vi "SQLite Get Calibration Kb Array.vi"(7 "Main":string="0", 8 "error in (no error)":errorcluster, 11 "VariableName":string) -> (0 "error out":errorcluster, 1 "Calibration Unit":T4, 2 "Calibration":T1, 3 "Calibration Kb&Volts":T2, 4 "XY":cluster{"X":dbl[], "Y":dbl[]}, 5 "Result Set 2":string[][](table) caption="Result Set (from first statement with results)", 6 "number":dbl[][](array[numeric]))   [LabVIEW 2017, in "SQLite.lvclass"]
doc: "从数据库读取多点校准数据，自动计算Kb的值。\n2015-11-03 15:56:09\n蒋松\njiangsong@outlook.com"
uses:
  SQLite.lvclass
  Calibration Unit.ctl
  Calibration Kb and Volt.ctl
  Calibration K and b Array.ctl
  Calibration K and b.ctl
  SQLiteFileName.ctl
  TabelFullName.ctl
  <vilib>/Utility/error.llb/Trim Whitespace.vi
  <userlib>/_MGI/1D Array/MGI Calculate Array Differences/MGI Calculate Array Differences (DBL[]).vi
  <userlib>/LabSQL/LabSQL.lvlib
  <userlib>/sushu/sushu.lvlib
panel:
  out "Select SQL CMD":string
  in  "error in (no error) 2":errorcluster
  out "y(i)=x(i)-x(i-1) 2":dbl[](array[numeric]) format="%.2f"
  out "y(i)=x(i)-x(i-1)":dbl[](array[numeric]) format="%.2f"
  out "x/y":dbl[](array[numeric])
  in  "OK":bool
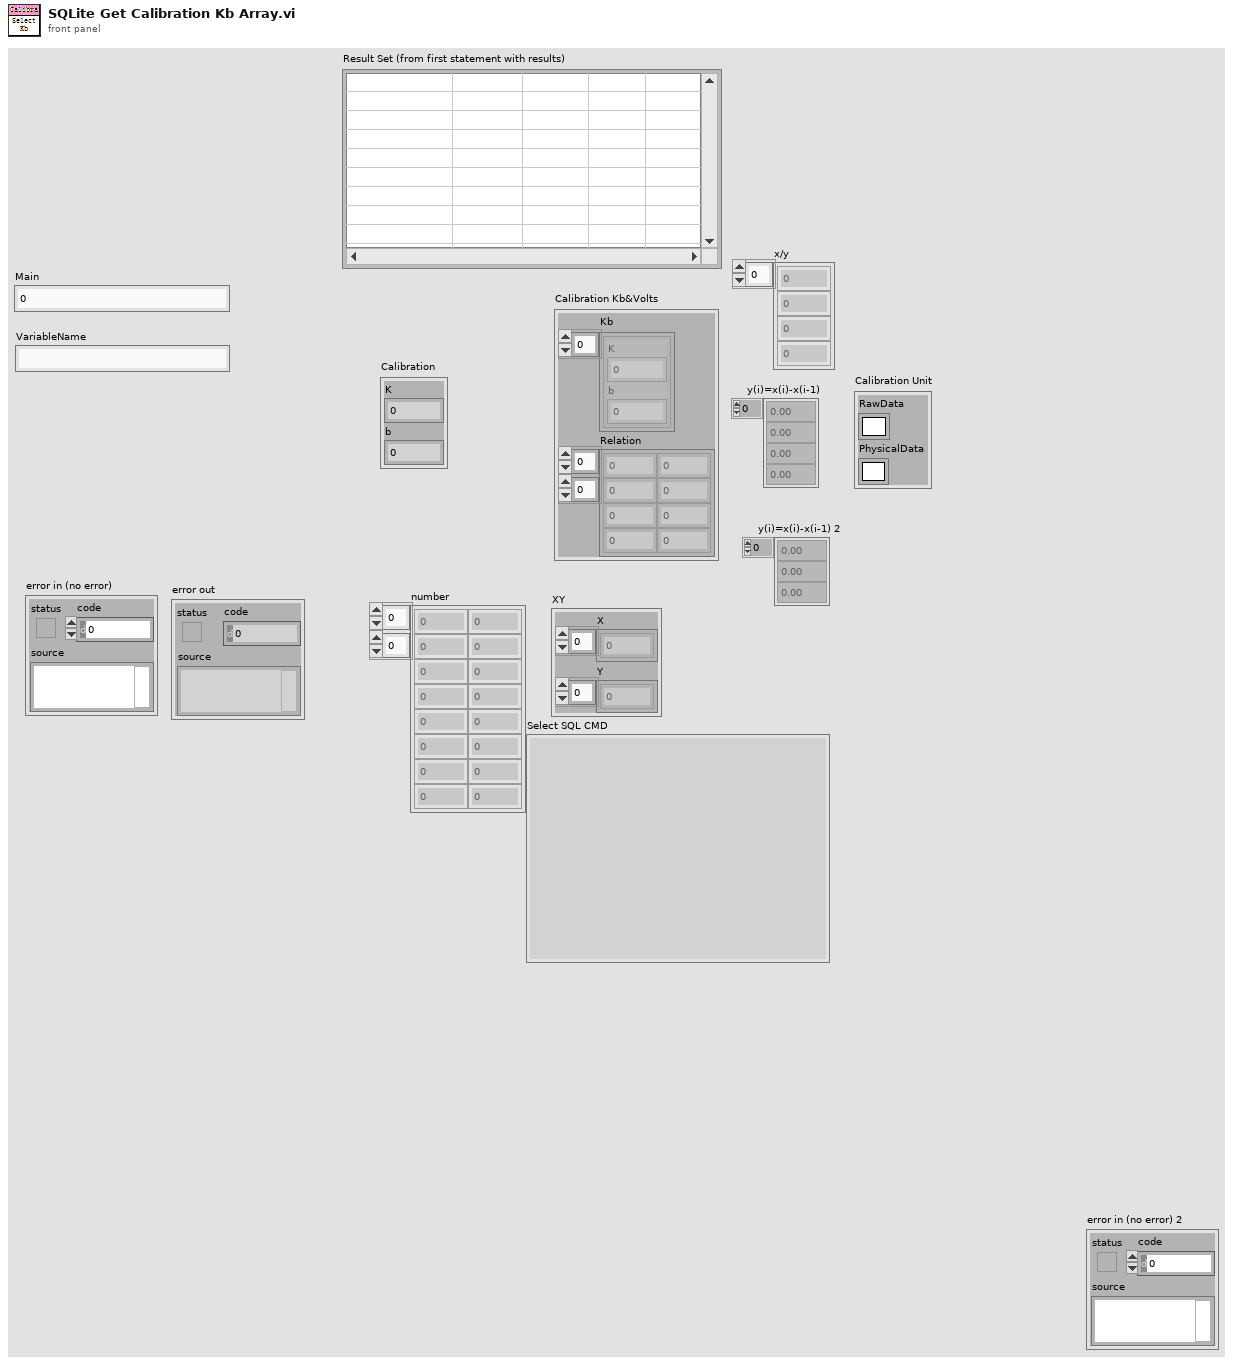
[diagram p1: front panel]
types:
  T1 = typedef "SQLite.lvclass/Calibration K and b.ctl" = cluster{"K":dbl, "b":dbl}
  T2 = typedef "SQLite.lvclass/Calibration Kb and Volt.ctl" = cluster{"Kb":T3, "Relation":dbl[][]}
  T3 = typedef "SQLite.lvclass/Calibration K and b Array.ctl" = T1[]
  T4 = typedef "SQLite.lvclass/Calibration Unit.ctl" = cluster{"RawData":string, "PhysicalData":string}
  T5 = typedef "SQLite.lvclass/TabelFullName.ctl" = string
  T6 = typedef "SQLite.lvclass/SQLiteFileName.ctl" = string
  T7 = enum16{"Other", "SQL2008", "SQLite", "Access", "MySQL"}
  T8 = cluster{"Current VI Reference":refnum<vi>, "Close Panel on Exit?":bool}
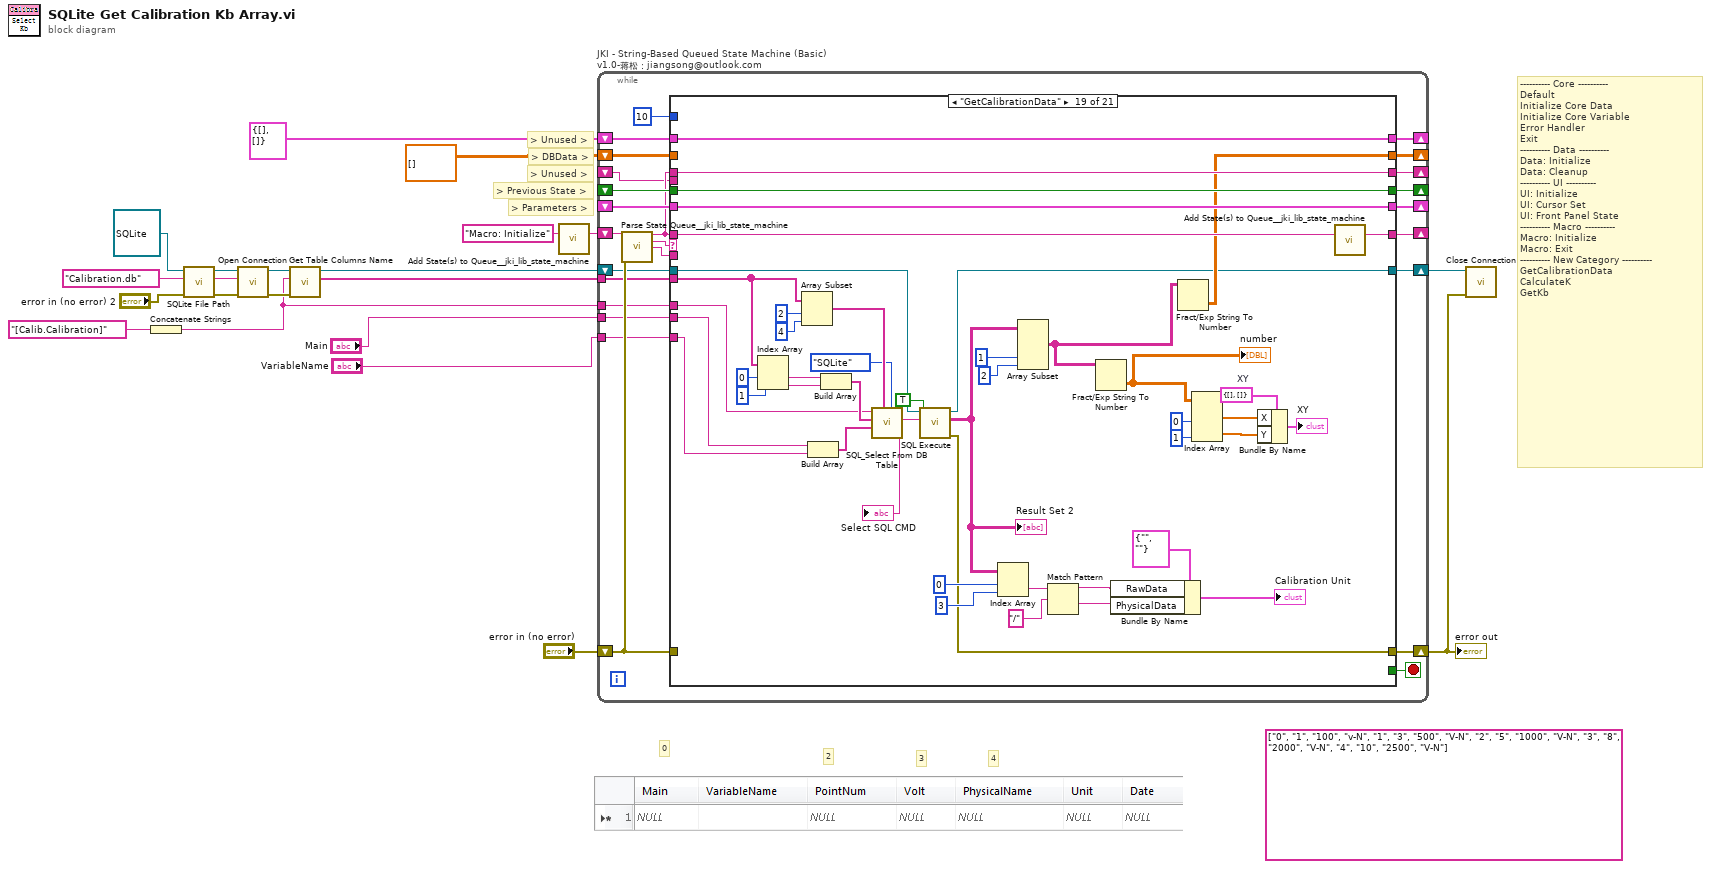
[diagram p0: block diagram]
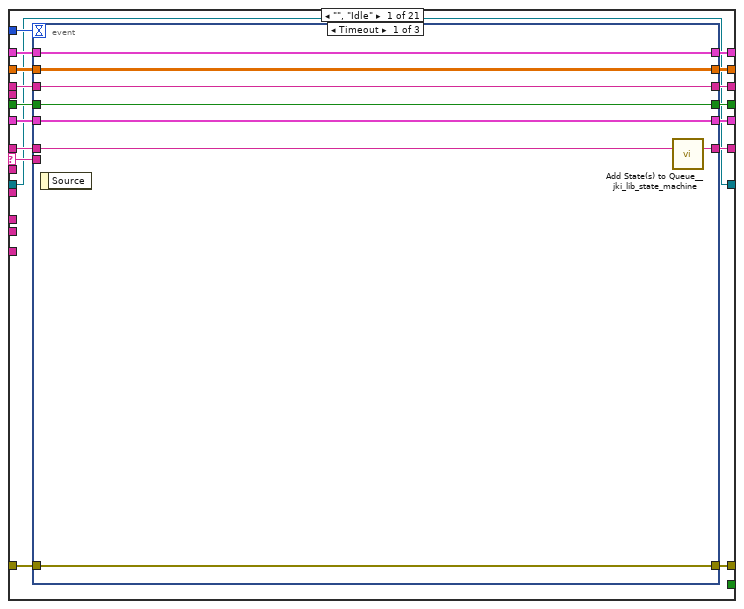
[diagram p2: hidden frame]
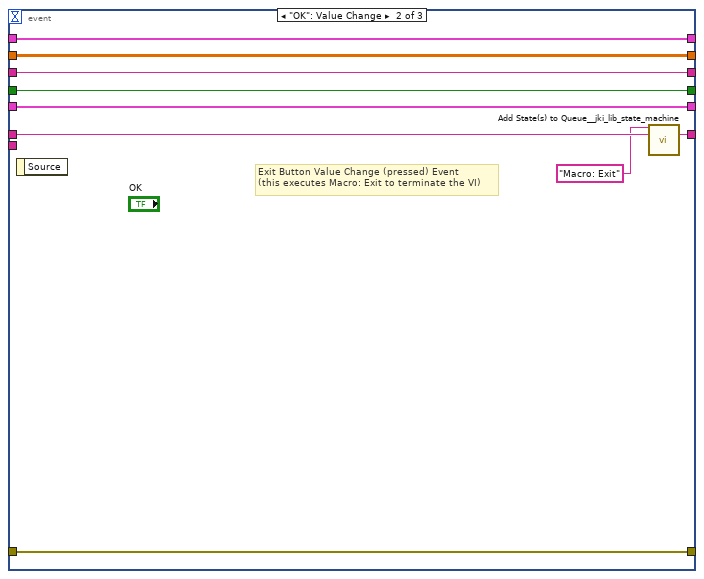
[diagram p3: hidden frame]
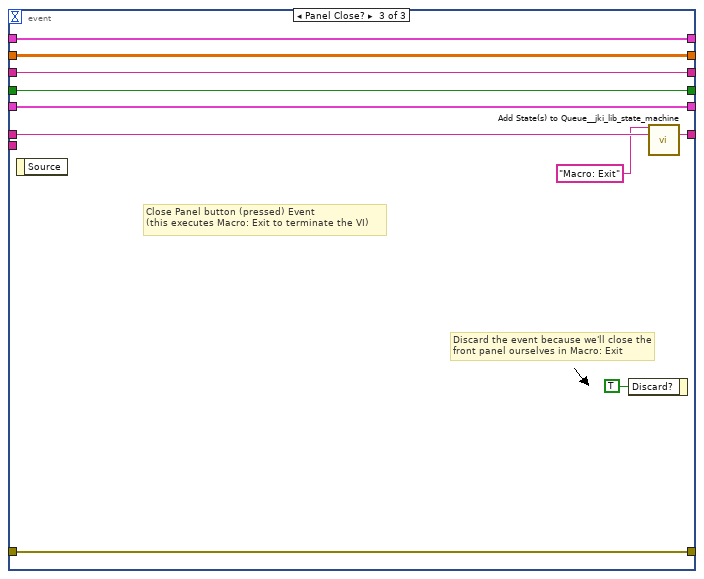
[diagram p4: hidden frame]
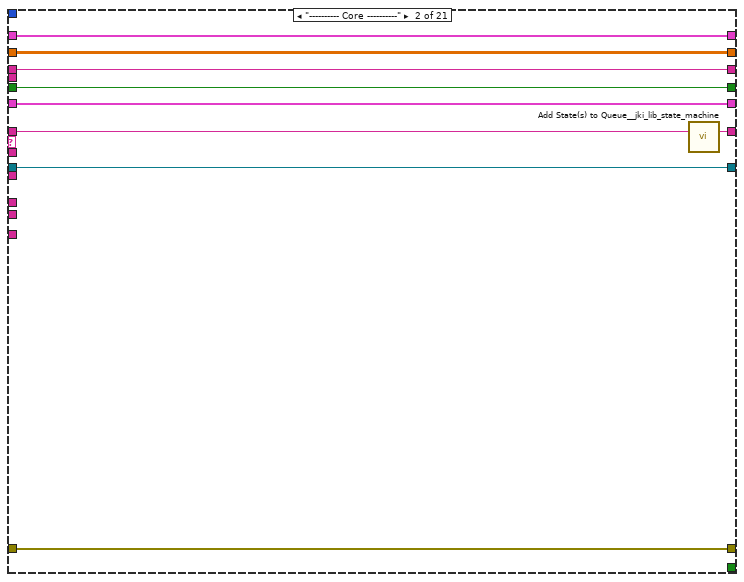
[diagram p5: hidden frame]
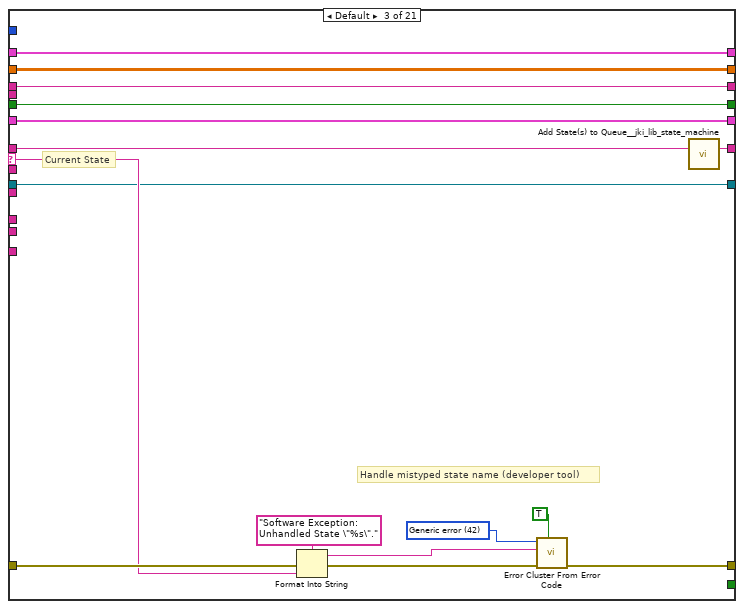
[diagram p6: hidden frame]
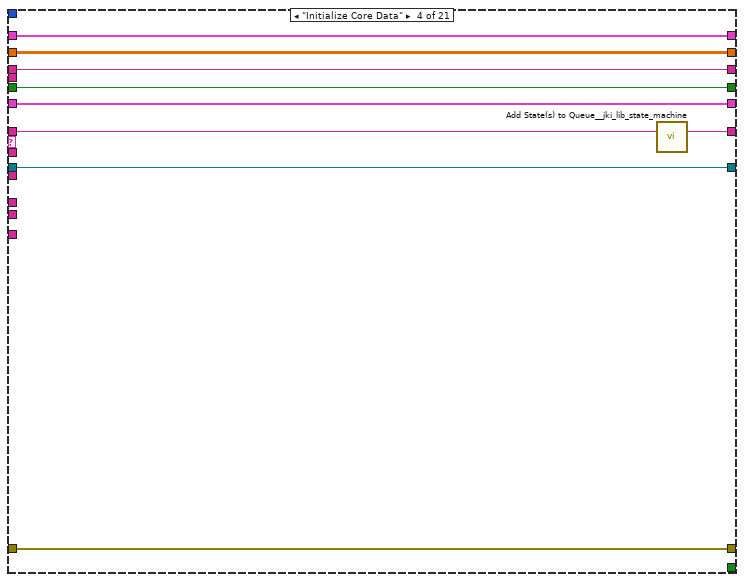
[diagram p7: hidden frame]
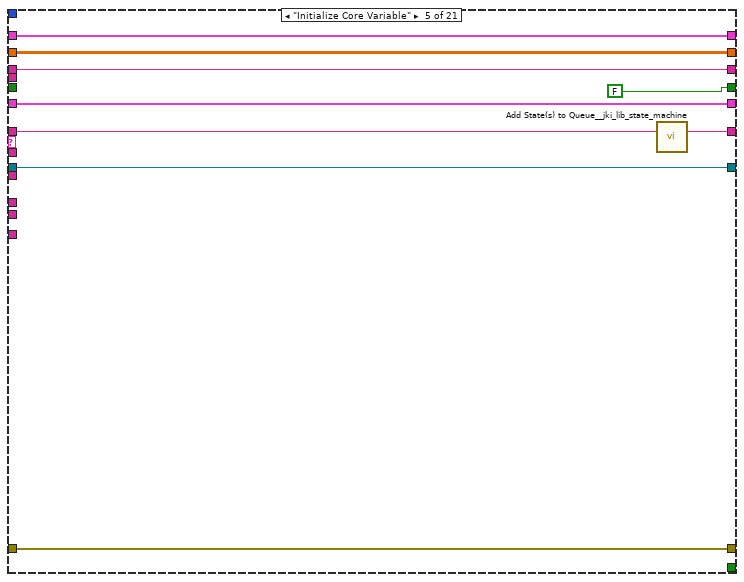
[diagram p8: hidden frame]
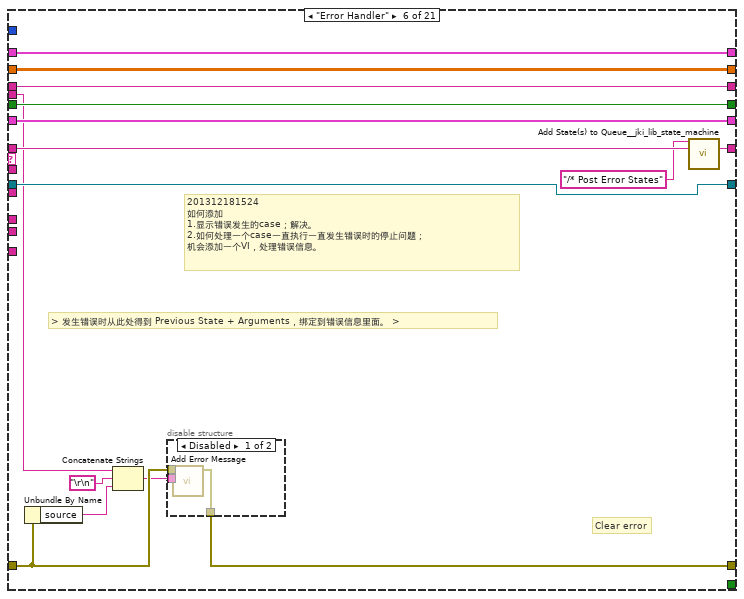
[diagram p9: hidden frame]
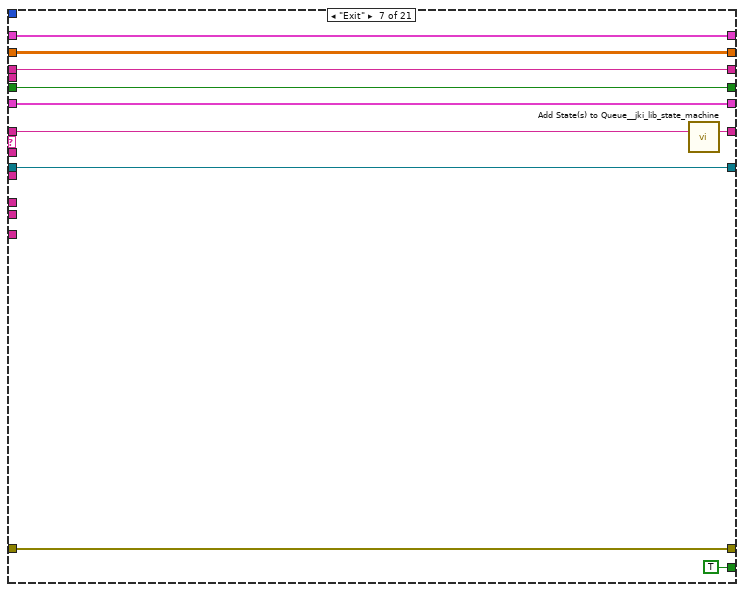
[diagram p11: hidden frame]
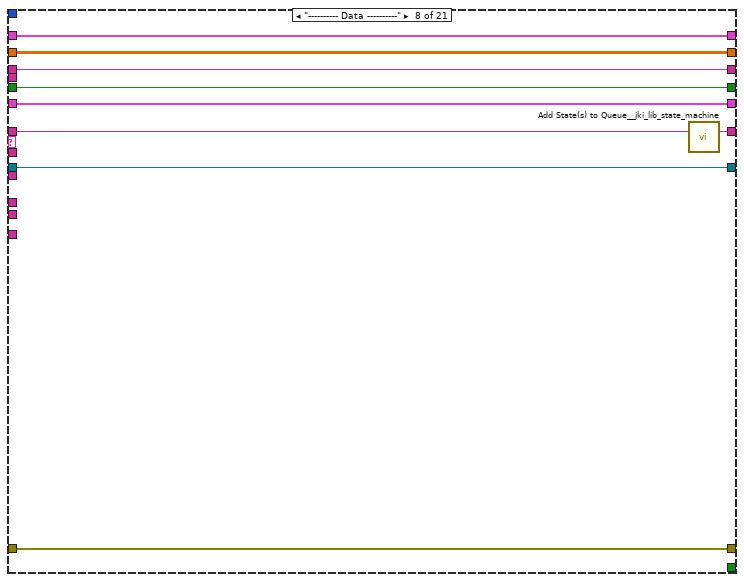
[diagram p12: hidden frame]
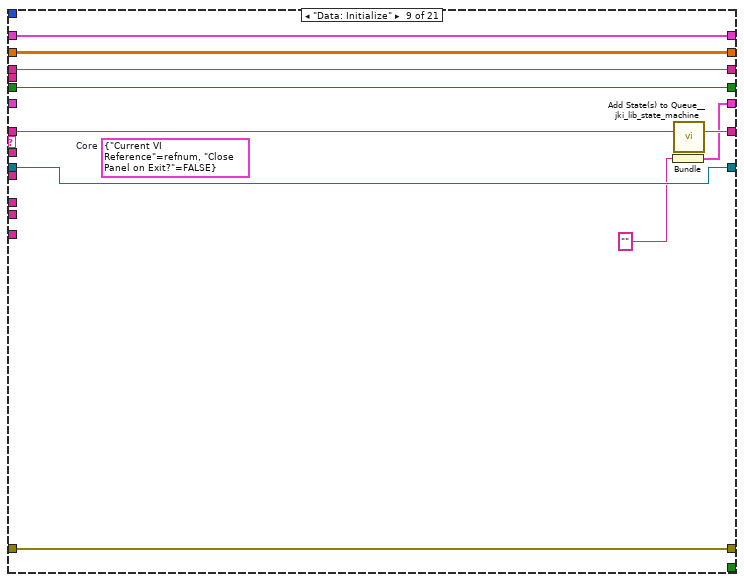
[diagram p13: hidden frame]
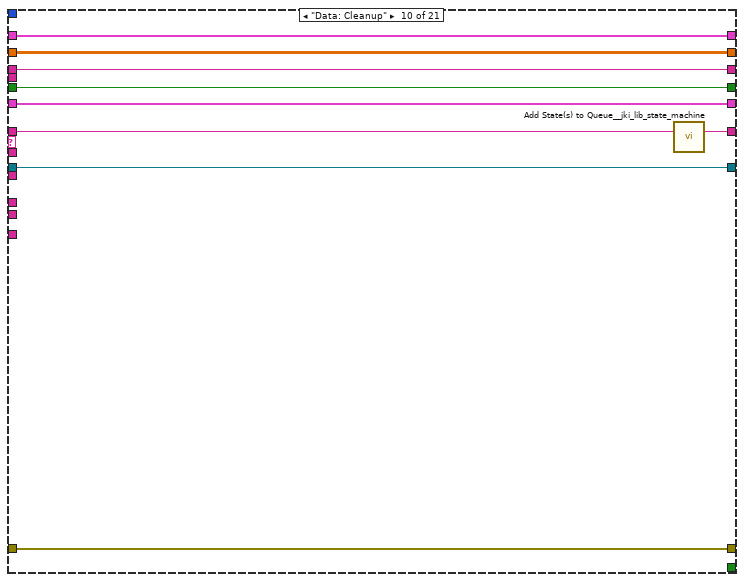
[diagram p14: hidden frame]
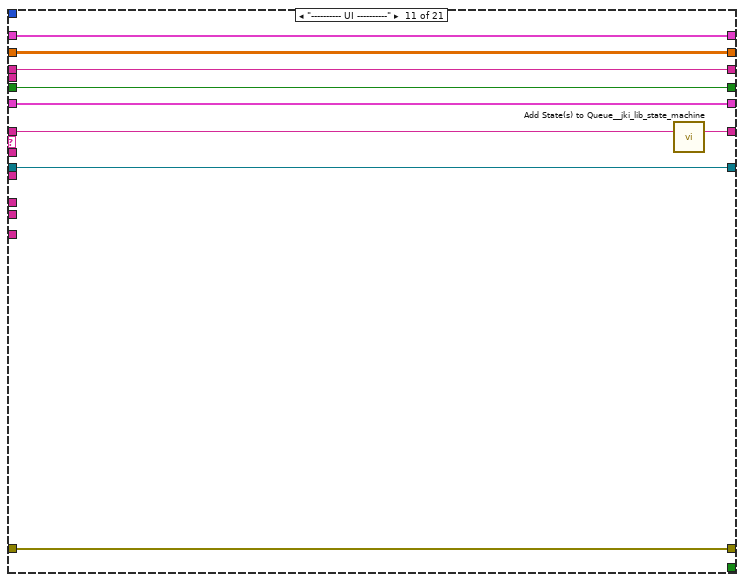
[diagram p15: hidden frame]
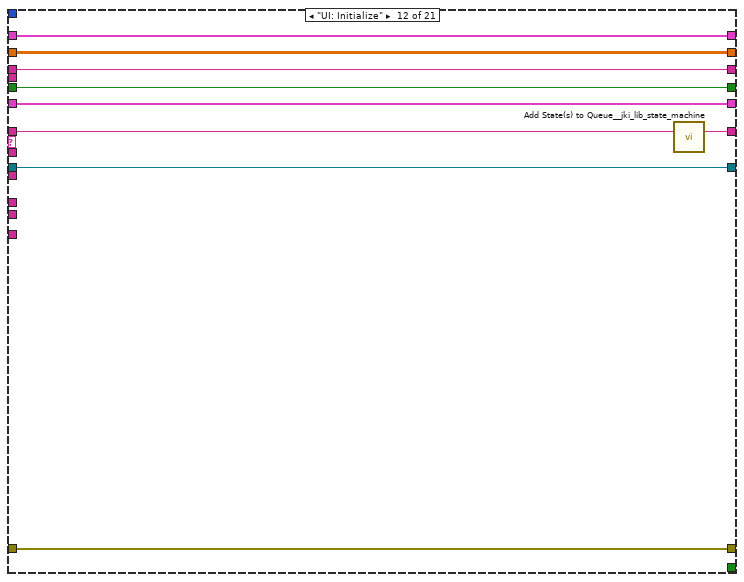
[diagram p16: hidden frame]
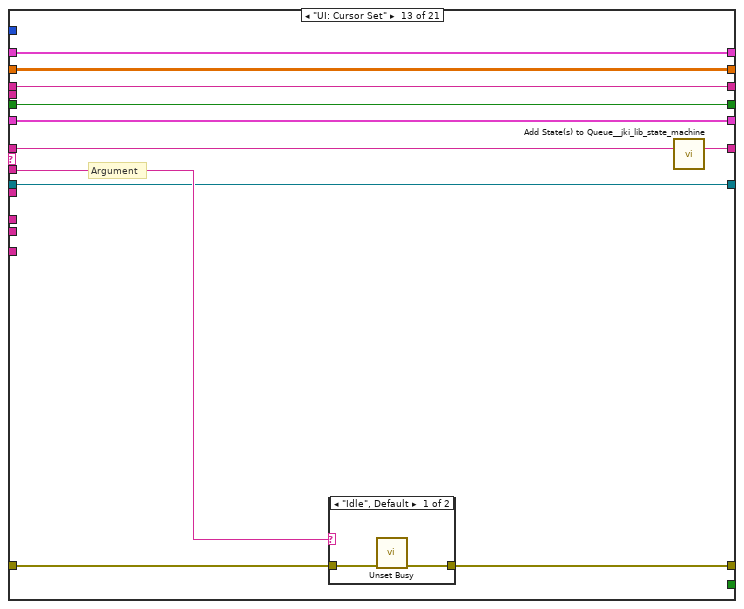
[diagram p17: hidden frame]
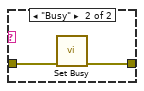
[diagram p18: hidden frame]
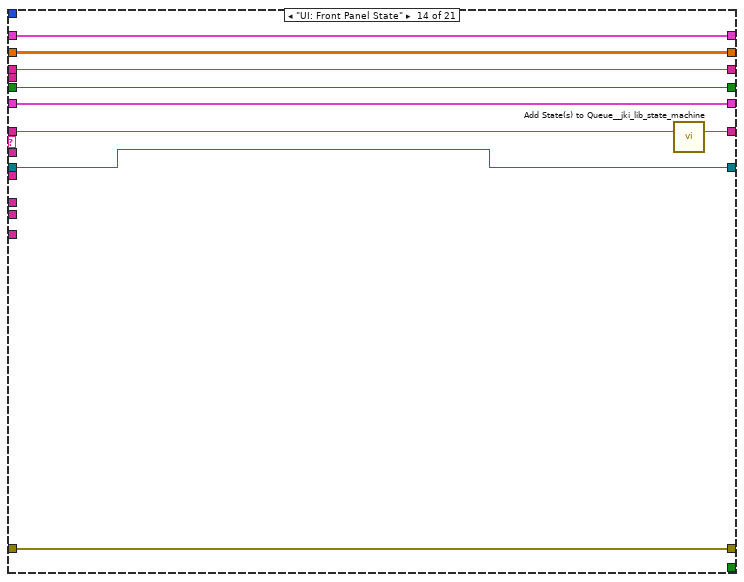
[diagram p19: hidden frame]
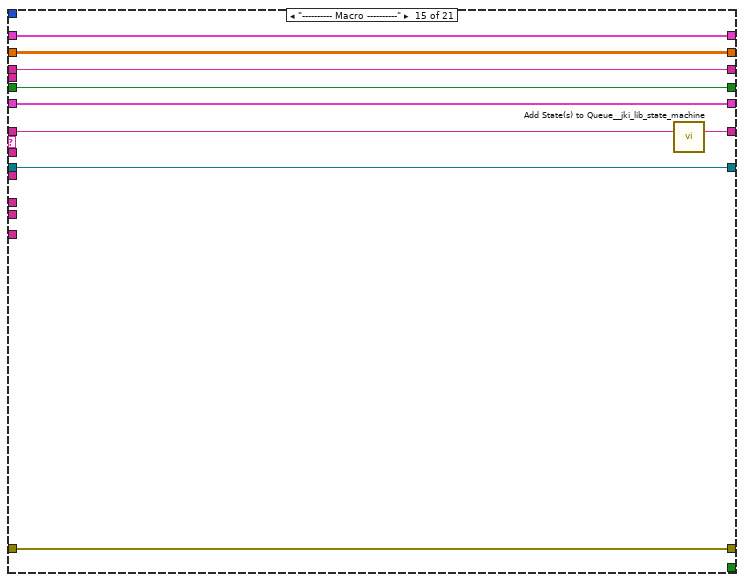
[diagram p20: hidden frame]
diagram:
  (unwired) string[][] [["0", "1", "100", "v-N"], ["1", "3", "500", "V-N"], ["2", "5", "1000", "V-N"], ["3", "8", "2000", "V-N"], ["4", "10", "2500", "V-N"]] ("Result Set 2")
  # "3"
  # "0"
  # "> Parameters >"
  # "> Previous State >"
  # "> Unused >"
  # "> DBData >"
  # "> Unused >"
  # "---------- Core ----------\nDefault\nInitialize Core Data\nInitialize Core Variable\nError Handler\nExit\n---------- Data ----------\nData: Initialize\nData: Cleanup\n---------- UI ----------\nUI: Initialize\nUI: Cursor Set\nUI: Front Panel State\n---------- Macro ----------\nMacro: Initialize\nMacro: Exit\n---------- New Category ----------\nGetCalibrationData\nCalculateK\nGetKb"
  # "2"
  # "4"
  n1 = Concatenate Strings(T5 "[Calib.Calibration]" ("TabelFullName")) -> (w4:string)
  n2 = call "SQLite File Path.vi"("error in (no error)"="error in (no error) 2", "SQLiteFileName"=T6 "Calibration.db", "SQLite in"=refnum<class "SQLite.lvclass"> refnum ("SQLite.lvclass")) -> ("error out"=w15:errorcluster, "string"=w10:string, "SQLite out"=w12:refnum<class "SQLite.lvclass">)  [unwired: 6 in]
  n3 = call-dynamic "Open Connection.vi"("error in (no error)"=w15, "ConnectionString"=w10, "HostDB in"=w12) -> ("error out"=w9:errorcluster, "HostDB out"=w8:refnum<class "SQLite.lvclass">)  [unwired: 7 in]
  n4 = call-dynamic "Get Table Columns Name.vi"("error in (no error)"=w9, "TableName"=w4, "HostDB in"=w8) -> ("ColunmsList"=w5:string[], "HostDB out"=w6:refnum<class "SQLite.lvclass">)  [unwired: 4 in, 3 out]
  n5 = call <vilib>:"Add State(s) to Queue__jki_lib_state_machine.vi"("State(s) in (\"\")"="Macro: Initialize") -> ("States Out"=w21:string)  [unwired: 14 in]
  n6 = while "JKI - String-Based Queued State Machine (Basic) v1.0-蒋松：jiangsong@outlook.com" {
    shift-right: [w44] -> w2
    shift-left: "error in (no error)" -> [w40]
    shift-right: [w43] -> _
    shift-left: w21 -> [w31]
    shift-right: [w36] -> _
    shift-left: dbl[][] [] ("number") -> [w38]
    shift-right: [w37] -> _
    shift-left: T2 {"Kb"=[], "Relation"=[]} ("Calibration") -> [w39]
    shift-right: [w32] -> _
    shift-left: _ -> [w35]
    shift-right: [w33] -> _
    shift-left: _ -> [w24]
    shift-right: [w34] -> _
    shift-left: _ -> [w22]
    tunnel: w5 -> [w30]
    tunnel: w4 -> [w29]
    tunnel: "Main" -> [w28]
    tunnel: "VariableName" -> [w27]
    shift-right: [w25] -> w3
    shift-left: w6 -> [w26]
    stop <- w42 stop-if-true
    n7 = call <vilib>:"Parse State Queue__jki_lib_state_machine.vi"("State Queue"=w31, "Error In (no error)"=w40) -> ("Remaining States"=w23:string, "Current State"=w46:string, "Arguments"=w45:string)  [unwired: 10 in, 1 out]
    n8 = case shown="\"GetCalibrationData\"" w46 {
      selector: w46 -> [w49 _ w101 _ _ _ _ _ _ _ _ _ _ _ _ _ _ _ _ _ _]
      tunnel: w23 -> [w63 w99 w115 w124 w133 w148 w161 w170 w180 w189 w198 w207 w218 w231 w240 w250 w260 w269 w314 w337 w375]
      tunnel: w45 -> [_ _ _ _ _ _ _ _ _ _ _ _ w212 _ _ _ _ _ _ _ _]
      tunnel: [w61 w97 w102 w119 w131 w135 w154 w164 w175 w181 w192 w201 w210 w223 w234 w244 w255 w264 w274 w331 w356] -> w44
      tunnel: w40 -> [w60 w97 w103 w119 w131 w138 w154 w164 w175 w181 w192 w201 w211 w223 w234 w244 w255 w264 _ w331 w356]
      tunnel: [w62 w98 w114 w123 w132 w147 w160 w169 w179 w188 w197 w206 w217 w230 w239 w249 w259 w268 w313 w336 w374] -> w43
      tunnel: [_ _ _ _ _ _ TRUE _ _ _ _ _ _ _ _ _ _ _ _ _ _] -> w42
      tunnel: 10 ("Timeout") -> [w59 _ _ _ _ _ _ _ _ _ _ _ _ _ _ _ _ _ _ _ _]
      tunnel: w39 -> [w58 w96 w113 w122 w127 w146 w159 w168 w178 w187 w196 w205 w216 w229 w238 w248 w258 w267 w312 w321 w373]
      tunnel: w38 -> [w57 w95 w112 w121 w129 w145 w158 w167 w177 w186 w195 w204 w215 w228 w237 w247 w257 w266 _ w320 w355]
      tunnel: [w56 w96 w113 w122 w127 w146 w159 w168 w178 w187 w196 w205 w216 w229 w238 w248 w258 w267 w312 w321 w373] -> w37
      tunnel: [w55 w95 w112 w121 w129 w145 w158 w167 w177 w186 w195 w204 w215 w228 w237 w247 w257 w266 w296 w320 w355] -> w36
      tunnel: w23 -> [w53 w94 w111 w120 w125 w144 w157 w166 w176 w185 w194 w203 w214 w227 w236 w246 w256 w265 w311 w335 w372]
      tunnel: w24 -> [w52 w92 w110 w118 _ w141 w153 w163 w173 w183 w191 w200 w209 w225 w233 w242 w253 w262 w309 w333 w370]
      tunnel: w35 -> [w50 w93 w109 w116 w130 w136 w156 w165 _ w184 w193 w202 w213 w226 w235 w245 w254 w263 w310 w334 w371]
      tunnel: [w54 w94 w111 w120 w125 w144 w157 w166 w176 w185 w194 w203 w214 w227 w236 w246 w256 w265 w311 w335 w372] -> w34
      tunnel: [w48 w92 w110 w118 FALSE w141 w153 w163 w173 w183 w191 w200 w209 w225 w233 w242 w253 w262 w309 w333 w370] -> w33
      tunnel: [w51 w93 w109 w116 w130 w136 w156 w165 w174 w184 w193 w202 w213 w226 w235 w245 w254 w263 w310 w334 w371] -> w32
      tunnel: w30 -> [_ _ _ _ _ _ _ _ _ _ _ _ _ _ _ _ _ _ w297 _ _]
      tunnel: w29 -> [_ _ _ _ _ _ _ _ _ _ _ _ _ _ _ _ _ _ w300 _ _]
      tunnel: w28 -> [_ _ _ _ _ _ _ _ _ _ _ _ _ _ _ _ _ _ w299 _ _]
      tunnel: w27 -> [_ _ _ _ _ _ _ _ _ _ _ _ _ _ _ _ _ _ w298 _ _]
      tunnel: w26 -> [w47 w91 w100 w117 w128 w139 w152 w162 w172 w182 w190 w199 w208 w224 w232 w241 w252 w261 w276 w332 w369]
      tunnel: [w47 w91 w100 w117 w128 w139 w152 w162 w172 w182 w190 w199 w208 w224 w232 w241 w252 w261 w275 w332 w369] -> w25
      tunnel: w22 -> [_ _ _ _ _ w134 _ _ _ _ _ _ _ _ _ _ _ _ _ _ _]
      frame "", "Idle" {
        n9 = event shown="[0] Timeout" {
          selector: _ -> [_ _ _]
          dyn-events: _ -> [_ _ _]
          timeout: w59 -> [_ _ _]
          tunnel: w63 -> [w71 w80 w90]
          tunnel: [w70 w79 w89] -> w62
          tunnel: [w69 w78 w88] -> w61
          tunnel: w60 -> [w69 w78 w88]
          tunnel: w58 -> [w68 w77 w87]
          tunnel: w57 -> [w67 w76 w86]
          tunnel: [w68 w77 w87] -> w56
          tunnel: [w67 w76 w86] -> w55
          tunnel: [w66 w75 w85] -> w54
          tunnel: w53 -> [w66 w75 w85]
          tunnel: w52 -> [w64 w72 w81]
          tunnel: [w65 w74 w84] -> w51
          tunnel: w50 -> [w65 w74 w84]
          tunnel: w49 -> [_ _ _]
          tunnel: [w64 w72 w81] -> w48
          event Timeout {
            n10 = event-data() -> ()  [unwired: 1 in, 1 out]
            n11 = call <vilib>:"Add State(s) to Queue__jki_lib_state_machine.vi"("State(s) in (\"\")"=w71) -> ("States Out"=w70:string)  [unwired: 14 in]
          }
          event "OK": Value Change {
            # "Exit Button Value Change (pressed) Event\n(this executes Macro: Exit to terminate the VI)"
            n12 = event-data() -> ()  [unwired: 1 in, 1 out]
            n13 = call <vilib>:"Add State(s) to Queue__jki_lib_state_machine.vi"("State(s) in Front (\"\")"="Macro: Exit", "State(s) in (\"\")"=w80) -> ("States Out"=w79:string)  [unwired: 13 in]
          }
          event Panel Close? {
            # "Discard the event because we'll close the front panel ourselves in Macro: Exit"
            # "Close Panel button (pressed) Event\n(this executes Macro: Exit to terminate the VI)"
            n14 = event-data() -> ()  [unwired: 1 in, 1 out]
            n15 = event-data("Discard?"=TRUE) -> ()  [unwired: 1 in, 1 out]
            n16 = call <vilib>:"Add State(s) to Queue__jki_lib_state_machine.vi"("State(s) in Front (\"\")"="Macro: Exit", "State(s) in (\"\")"=w90) -> ("States Out"=w89:string)  [unwired: 13 in]
          }
        }
      }
      frame "---------- Core ----------" {
        n17 = call <vilib>:"Add State(s) to Queue__jki_lib_state_machine.vi"("State(s) in (\"\")"=w99) -> ("States Out"=w98:string)  [unwired: 14 in]
      }
      frame Default {
        w105 = 42 items=["No error", "Argument error", "Memory is full", "Out of zone", "End of file", "File already open", "Generic file I/O error", "File not found", "File permission error", "Disk is full", "Duplicate path", "Too many files open", "System feature not enabled", "Resource file not found", "Cannot add resource", "Resource not found", "Image not found", "Image memory error", "Pen does not exist", "Config type invalid", "Config token not found", "Config parse error", "Config memory error", "Bad external code format", "Bad external code offset", "External code not present", "Null window", "Destroy window error", "Null menu", "Print aborted", "Bad print record", "Print driver error", "Windows error during printing", "Memory error during printing", "Print dialog error", "Generic print error", "Invalid device refnum", "Device not found", "Device parameter error", "Device unit error", "Cannot open device", "Device call aborted", "Generic error", "Cancelled by user", "Object ID too low", "Object ID too high", "Object not in heap", "Unknown heap", "Unknown object (invalid DefProc)", "Unknown object (DefProc not in table)", "Message out of range", "Invalid (null) method", "Unknown message", "Manager call not supported", "Bad address", "Network operation in progress", "Network operation timed out", "Connection is busy", "Network attribute not supported", "Network error", "Address in use", "System out of memory", "Connection aborted", "Connection refused", "Not connected", "Already connected", "Connection closed", "Initialization error (interapplication manager)", "Bad occurrence", "Wait on unbound occurrence handler", "Occurrence queue overflow", "Datalog type conflict", "Unused", "Unrecognized type (interapplication manager)", "Memory corrupt", "Failed to make temporary DLL", "Old CIN version", "Drag socket not found", "Failed to load drop-object", "Failed to register OLE object", "Failed to release OLE object", "Format specifier type mismatch", "Unknown format specifier", "Too few format specifiers", "Too many format specifiers", "Scan failed", "Newer CIN version", "Error converting to variant", "Runtime menu error", "Password tampered", "Variant attribute not found", "Incompatible variant data type", "Event data is not available", "Event Store is not present", "Occurrence is not found", "Event Queue is not created", "Event info is not available", "Refnum passed is NULL", "Error retrieving Class GUID", "Error retrieving CoClass GUID", "Error retrieving TypeLib GUID.", "Bad built application magic bytes.", "Specific driver is different from the specific driver associated with the Logical Name.", "There is no session opened to the class driver.", "Max Error", "MAX - Error with config objects", "MAX - Error loading configuration", "MAX - Group not supported"]
        # "Current State"
        # "Handle mistyped state name (developer tool)"
        n18 = Format Into String(format string="Software Exception: Unhandled State \"%s\"." ("message"), error in=w103, w101) -> (resulting string=w106:string, error out=w107:errorcluster)  [unwired: 1 in]
        n19 = call <vilib>:"Error Cluster From Error Code.vi"("show call chain? (False)"=TRUE, "error in (no error)"=w107, "error message (\"\")"=w106, "error code (0)"=w105) -> ("error out"=w102:errorcluster)  [unwired: 5 in]
        n20 = call <vilib>:"Add State(s) to Queue__jki_lib_state_machine.vi"("State(s) in (\"\")"=w115) -> ("States Out"=w114:string)  [unwired: 14 in]
      }
      frame "Initialize Core Data" {
        n21 = call <vilib>:"Add State(s) to Queue__jki_lib_state_machine.vi"("State(s) in (\"\")"=w124) -> ("States Out"=w123:string)  [unwired: 14 in]
      }
      frame "Initialize Core Variable" {
        n22 = call <vilib>:"Add State(s) to Queue__jki_lib_state_machine.vi"("State(s) in (\"\")"=w133) -> ("States Out"=w132:string)  [unwired: 14 in]
      }
      frame "Error Handler" {
        # "> 发生错误时从此处得到 Previous State + Arguments，绑定到错误信息里面。 >"
        # "201312181524\n如何添加\n1.显示错误发生的case；解决。\n2.如何处理一个case一直执行一直发生错误时的停止问题；\n机会添加一个VI，处理错误信息。"
        # "Clear error"
        n23 = Unbundle By Name(w138) -> ("source"=w140:string)
        n24 = Concatenate Strings(w134, "\r\n", w140) -> (w137:string)
        n25 = disable-structure shown="Disabled" {
          disable-tunnel: w138 -> [w151 _]
          disable-tunnel: w137 -> [w150 _]
          disable-tunnel: [w149 _] -> w135
          frame Disabled {
            n26 = call <userlib>:"Add Error Message.vi"("ErrorMessages"=w150, "error in (no error)"=w151) -> ("error out"=w149:errorcluster)  [unwired: 9 in]
          }
          frame Enabled {
          }
        }
        n27 = call <vilib>:"Add State(s) to Queue__jki_lib_state_machine.vi"("State(s) in Front (\"\")"="/* Post Error States", "State(s) in (\"\")"=w148) -> ("States Out"=w147:string)  [unwired: 13 in]
      }
      frame "Exit" {
        n28 = call <vilib>:"Add State(s) to Queue__jki_lib_state_machine.vi"("State(s) in (\"\")"=w161) -> ("States Out"=w160:string)  [unwired: 14 in]
      }
      frame "---------- Data ----------" {
        n29 = call <vilib>:"Add State(s) to Queue__jki_lib_state_machine.vi"("State(s) in (\"\")"=w170) -> ("States Out"=w169:string)  [unwired: 14 in]
      }
      frame "Data: Initialize" {
        (unwired) T8 {"Current VI Reference"=refnum, "Close Panel on Exit?"=FALSE}  # Core
        n30 = Bundle("") -> (w174:cluster{string})  [unwired: 1 in]
        n31 = call <vilib>:"Add State(s) to Queue__jki_lib_state_machine.vi"("State(s) in (\"\")"=w180) -> ("States Out"=w179:string)  [unwired: 14 in]
      }
      frame "Data: Cleanup" {
        n32 = call <vilib>:"Add State(s) to Queue__jki_lib_state_machine.vi"("State(s) in (\"\")"=w189) -> ("States Out"=w188:string)  [unwired: 14 in]
      }
      frame "---------- UI ----------" {
        n33 = call <vilib>:"Add State(s) to Queue__jki_lib_state_machine.vi"("State(s) in (\"\")"=w198) -> ("States Out"=w197:string)  [unwired: 14 in]
      }
      frame "UI: Initialize" {
        n34 = call <vilib>:"Add State(s) to Queue__jki_lib_state_machine.vi"("State(s) in (\"\")"=w207) -> ("States Out"=w206:string)  [unwired: 14 in]
      }
      frame "UI: Cursor Set" {
        # "Argument"
        n35 = case shown="\"Idle\", Default" w212 {
          tunnel: w211 -> [w220 w222]
          tunnel: [w219 w221] -> w210
          frame "Idle", Default {
            n36 = call <vilib>:"Unset Busy.vi"("error in (no error)"=w220) -> ("error out"=w219:errorcluster)  [unwired: 10 in]
          }
          frame "Busy" {
            n37 = call <vilib>:"Set Busy.vi"("error in (no error)"=w222) -> ("error out"=w221:errorcluster)  [unwired: 9 in, 1 out]
          }
        }
        n38 = call <vilib>:"Add State(s) to Queue__jki_lib_state_machine.vi"("State(s) in (\"\")"=w218) -> ("States Out"=w217:string)  [unwired: 14 in]
      }
      frame "UI: Front Panel State" {
        n39 = call <vilib>:"Add State(s) to Queue__jki_lib_state_machine.vi"("State(s) in (\"\")"=w231) -> ("States Out"=w230:string)  [unwired: 14 in]
      }
      frame "---------- Macro ----------" {
        n40 = call <vilib>:"Add State(s) to Queue__jki_lib_state_machine.vi"("State(s) in (\"\")"=w240) -> ("States Out"=w239:string)  [unwired: 14 in]
      }
      frame "Macro: Initialize" {
        n41 = call <vilib>:"Add State(s) to Queue__jki_lib_state_machine.vi"("State(s) in Front (\"\")"="Data: Initialize\nInitialize Core Variable\nGetCalibrationData\nCalculateK\nGetKb\nMacro: Exit", "State(s) in (\"\")"=w250) -> ("States Out"=w249:string)  [unwired: 13 in]
      }
      frame "Macro: Exit" {
        n42 = call <vilib>:"Add State(s) to Queue__jki_lib_state_machine.vi"("State(s) in Front (\"\")"="Data: Cleanup\nExit", "State(s) in (\"\")"=w260) -> ("States Out"=w259:string)  [unwired: 13 in]
      }
      frame "---------- New Category ----------" {
        n43 = call <vilib>:"Add State(s) to Queue__jki_lib_state_machine.vi"("State(s) in (\"\")"=w269) -> ("States Out"=w268:string)  [unwired: 14 in]
      }
      frame "GetCalibrationData" {
        w291 = cluster{"X":dbl[], "Y":dbl[]} {"X"=[], "Y"=[]}  # XY
        n44 = Index Array(array=w297, index #1=0 ("index"), index #2=1 ("index")) -> (element #1=w304:string, element #2=w305:string)
        n45 = Array Subset(array=w297, index=2, length=4 ("index")) -> (w295:string[])
        n46 = Build Array(w299, w298) -> (w301:string[])
        n47 = Build Array(w304, w305) -> (w306:string[])
        n48 = call <userlib>:"SQL_Select From DB Table.vi"("DB Type"=T7."SQLite", "SelectedColumnsNameList"=w295, "ColumnsValue"=w301, "ColumnsNameList"=w306, "TableName"=w300) -> ("Select SQL CMD"=w277:string)  [unwired: 6 in]
        "Select SQL CMD" <- w277
        n49 = call-dynamic "SQL Execute.vi"("Return Data (T)"=TRUE, "Command Text"=w277, "HostDB in"=w276) -> ("error out"=w274:errorcluster, "Table Control"=w278:string[][], "HostDB out"=w275:refnum<class "SQLite.lvclass">)  [unwired: 4 in, 2 out]
        "Result Set 2" <- w278
        n50 = Index Array(array=w278, index (row)=0, index (col)=3 ("disabled index (col)")) -> (element=w282:string)
        n51 = Array Subset(array=w278, index (col)=1 ("length"), length (col)=2 ("length")) -> (w292:string[][])  [unwired: 2 in]
        n52 = Match Pattern(string=w282, regular expression="/") -> (before substring=w280:string, after substring=w279:string)  [unwired: 1 in, 2 out]
        n53 = Fract/Exp String To Number(string=w292) -> (number=w290:dbl[][])  [unwired: 3 in, 1 out]
        "number" <- w290
        n54 = Bundle By Name(cluster=T4 {"RawData"="", "PhysicalData"=""} ("Calibration Unit"), "RawData"=w280, "PhysicalData"=w279) -> (→"Calibration Unit":T4)
        n55 = Fract/Exp String To Number(string=w292) -> (number=w296:dbl[][])  [unwired: 3 in, 1 out]
        n56 = Index Array(array=w290, index (col) #1=0 ("disabled index (col)"), index (col) #2=1 ("index (col)")) -> (element #1=w287:dbl[], element #2=w286:dbl[])  [unwired: 2 in]
        n57 = Bundle By Name(cluster=w291, "X"=w287, "Y"=w286) -> (→"XY":cluster{"X":dbl[], "Y":dbl[]})
        n58 = call <vilib>:"Add State(s) to Queue__jki_lib_state_machine.vi"("State(s) in (\"\")"=w314) -> ("States Out"=w313:string)  [unwired: 14 in]
      }
      frame "CalculateK" {
        (unwired) dbl[][] [] ("number")
        w327 = 0 ("index")
        w328 = 1 ("length")
        # "Physical quantity"
        # "volt"
        n59 = Index Array(array=w320, index (col) #1=0 ("disabled index (col)"), index (col) #2=1 ("index (col)")) -> (element #1=w319:dbl[], element #2=w318:dbl[])  [unwired: 2 in]
        "y(i)=x(i)-x(i-1)" <- w318
        "y(i)=x(i)-x(i-1) 2" <- w319
        n60 = call-poly <userlib>:"MGI Calculate Array Differences.vi"("x(i)"=w319) -> ("y(i)=x(i)-x(i-1)"=w323:dbl[])  [unwired: 1 in]
        n61 = call-poly <userlib>:"MGI Calculate Array Differences.vi"("x(i)"=w318) -> ("y(i)=x(i)-x(i-1)"=w317:dbl[])  [unwired: 1 in]
        n62 = Delete From Array(array=w323, length=w328, index=w327) -> (array with subset deleted=w325:dbl[])  [unwired: 1 out]
        n63 = Delete From Array(array=w317, length=w328, index=w327) -> (array with subset deleted=w326:dbl[])  [unwired: 1 out]
        n64 = Divide(x=w326, y=w325) -> (x/y=w324:dbl[])
        "x/y" <- w324
        n65 = for {
          tunnel: w324 -> [w344] mode=indexing
          tunnel: w319 -> [w347] mode=indexing
          tunnel: w318 -> [w346] mode=indexing
          tunnel: [w343] -> _ mode=indexing
          shift-right: [w342] -> w322
          shift-left: T3 [] ("Kb Array") -> [w341]
          n66 = Multiply(x=w344, y=w347) -> (x*y=w345:dbl)
          n67 = Array Size(array=w341) -> (size(s)=w340:i32)
          n68 = Subtract(x=w346, y=w345) -> (x-y=w343:dbl)
          n69 = Bundle By Name(cluster=T1 {"K"=0.0, "b"=0.0} ("Calibration"), "K"=w344, "b"=w343) -> (w339:T1)
          n70 = Insert Into Array(array=w341, index=w340, new element=w339) -> (w342:T3)
        }
        n71 = Bundle By Name(cluster=w321, "Relation"=w320, "Kb"=w322) -> (→"Calibration Kb&Volts":T2)
        n72 = call <vilib>:"Add State(s) to Queue__jki_lib_state_machine.vi"("State(s) in (\"\")"=w337) -> ("States Out"=w336:string)  [unwired: 14 in]
      }
      frame "GetKb" {
        w368 = 2 ("y")
        w360 = 2 ("y")
        # "这个case仅仅适用2点校准\n2015-07-12 13:51:33"
        n73 = Array Size(array=w355) -> (size(s)=w357:i32[])
        n74 = Index Array(array=w357) -> (element=w358:i32)  [unwired: 1 in]
        n75 = Subtract(x=w358, y=w360) -> (x-y=w359:i32)
        n76 = Array Subset(array=w355, index (row)=w359, length (row)=w360) -> (w363:dbl[][])  [unwired: 2 in]
        n77 = Array Size(array=w363) -> (size(s)=w364:i32[])
        n78 = Index Array(array=w364, index=1) -> (element=w366:i32)
        n79 = Subtract(x=w366, y=w368) -> (x-y=w367:i32)
        n80 = Array Subset(array=w363, index (col)=w367, length (col)=w368) -> (w354:dbl[][])  [unwired: 2 in]
        n81 = Index Array(array=w354, index (col) #1=1 ("disabled index (col)"), index (col) #2=0 ("index (col)")) -> (element #1=w351:dbl[], element #2=w350:dbl[])  [unwired: 2 in]
        n82 = call "Calculate K and b.vi"("X"=w350, "Y"=w351) -> ("b"=w348:dbl, "K"=w349:dbl)  [unwired: 8 in]
        n83 = Bundle By Name(cluster=T1 {"K"=0.0, "b"=0.0} ("Calibration"), "K"=w349, "b"=w348) -> (→"Calibration":T1)
        n84 = call <vilib>:"Add State(s) to Queue__jki_lib_state_machine.vi"("State(s) in (\"\")"=w375) -> ("States Out"=w374:string)  [unwired: 14 in]
      }
    }
  }
  "error out" <- w2
  n85 = call-dynamic "Close Connection.vi"("error in (no error)"=w2, "HostDB in"=w3) -> ()  [unwired: 8 in, 2 out]
